vi "RANGE Meter Bank Select 3.vi"(8 "Error In":errorcluster, 10 "Meter Data":T2, 11 "Meter Select Bank 3":T1) -> (0 "Error Out":errorcluster, 2 "Unit ID":string, 3 "VISA Refnum out":refnum<visa-resource-name>)   [LabVIEW 2016]
uses:
  Type Definitions/RANGE DAQ Data Four Meters.ctl
  Type Definitions/RANGE DAQ Data.ctl
  Drivers/Omega FMA-1600A Series Gas Flow Meter/Type Definitions/FMA1600A Gas Type.ctl
  Drivers/Omega FMA-1600A Series Gas Flow Meter/Type Definitions/FMA1600A Units String.ctl
  Type Definitions/RANGE GAS Data.ctl
  Type Definitions/RANGE Panel Data.ctl
  Type Definitions/RANGE Meter Selector 5-6.ctl
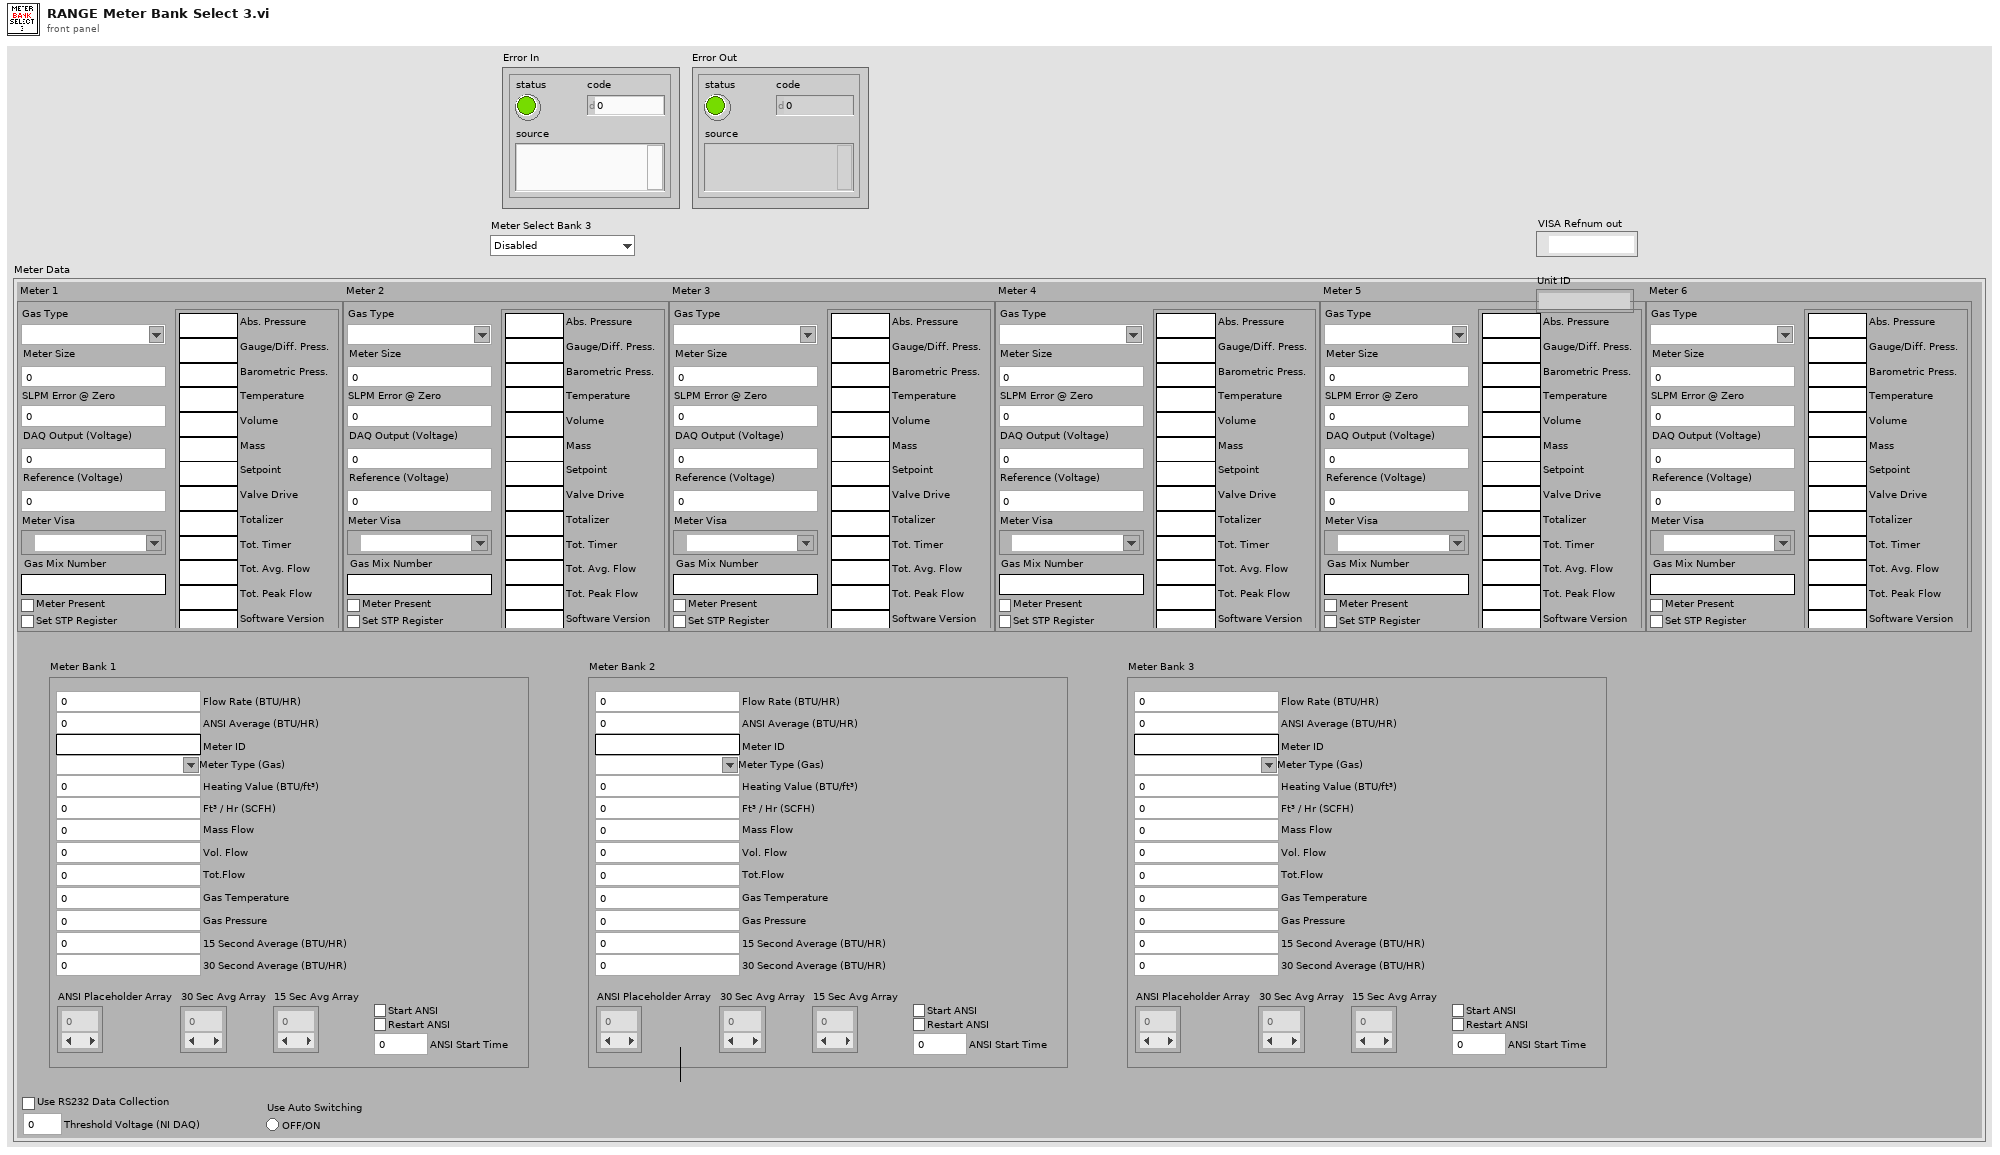
[diagram p1: front panel]
types:
  T1 = typedef "RANGE Meter Selector 5-6.ctl" = enum16{"Disabled", "Meter 5", "Meter 6", "Auto"}
  T2 = typedef "RANGE DAQ Data Four Meters.ctl" = cluster{"Meter 1":T3, "Meter 2":T3, "Meter 3":T3, "Meter 4":T3, "Meter 5":T3, "Meter 6":T3, "Meter Bank 1":T6, "Meter Bank 2":T6, "Meter Bank 3":T6, "Threshold Voltage (NI DAQ)":dbl, "Use RS232 Data Collection":bool, "Use Auto Switching":bool}
  T3 = typedef "RANGE DAQ Data.ctl" = cluster{"Meter Size":dbl, "DAQ Output (Voltage)":dbl, "Reference (Voltage)":dbl, "Meter Present":bool, "Meter Visa":refnum<visa-resource-name>, "Gas Type":T4, "SLPM Error @ Zero":dbl, "Gas Mix Number":string, "Set STP Register":bool, "Measurement Units":T5}
  T4 = typedef "FMA1600A Gas Type.ctl" = string
  T5 = typedef "FMA1600A Units String.ctl" = cluster{"Abs. Pressure":string, "Gauge/Diff. Press.":string, "Barometric Press.":string, "Temperature":string, "Volume":string, "Mass":string, "Setpoint":string, "Valve Drive":string, "Totalizer":string, "Tot. Timer":string, "Tot. Avg. Flow":string, "Tot. Peak Flow":string, "Software Version":string}
  T6 = typedef "RANGE GAS Data.ctl" = cluster{"Flow Rate (BTU/HR)":dbl, "ANSI Placeholder Array":dbl[], "15 Sec Avg Array":dbl[], "30 Sec Avg Array ":dbl[], "ANSI Average (BTU/HR)":dbl, "Panel Data":T7, "Start ANSI":bool, "ANSI Start Time":dbl, "Restart ANSI":bool, "Meter ID":string}
  T7 = typedef "RANGE Panel Data.ctl" = cluster{"Meter Type (Gas)":T4, "Heating Value (BTU/ft³)":dbl, "Ft³ / Hr (SCFH)":dbl, "15 Second Average (BTU/HR)":dbl, "30 Second Average (BTU/HR)":dbl, "Mass Flow":dbl, "Vol. Flow":dbl, "Gas Temperature":dbl, "Gas Pressure":dbl, "Tot.Flow":dbl}
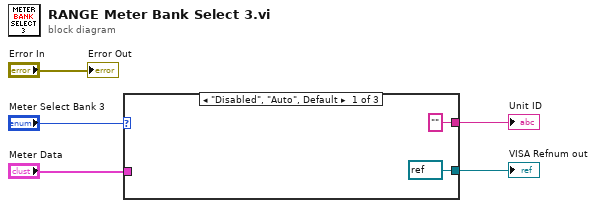
[diagram p0: block diagram]
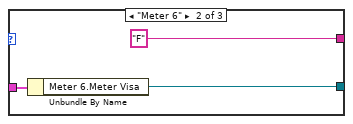
[diagram p2: hidden frame]
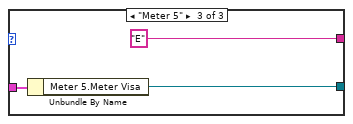
[diagram p3: hidden frame]
diagram:
  n1 = case shown="\"Disabled\", \"Auto\", Default" "Meter Select Bank 3" {
    tunnel: ["" "F" "E"] -> w3
    tunnel: "Meter Data" -> [_ w9 w12]
    tunnel: [refnum<visa-resource-name> refnum ("Meter Visa") w8 w11] -> w4
    frame "Disabled", "Auto", Default {
    }
    frame "Meter 6" {
      n2 = Unbundle By Name(w9) -> ("Meter 6.Meter Visa"=w8:refnum<visa-resource-name>)
    }
    frame "Meter 5" {
      n3 = Unbundle By Name(w12) -> ("Meter 5.Meter Visa"=w11:refnum<visa-resource-name>)
    }
  }
  "VISA Refnum out" <- w4
  "Unit ID" <- w3
  "Error Out" <- "Error In"
